vi "Dequeue.vi"(8 "error in (no error)":errorcluster caption="错误输入（无错误）", 11 "Queue 输入":refnum<class "Queue.lvclass"> caption="DNL_LabVIEW Object in") -> (0 "error out":errorcluster caption="错误输出", 2 "Item":variant, 3 "Queue 输出":refnum<class "Queue.lvclass"> caption="DNL_LabVIEW Object out")   [LabVIEW 2012, in "Queue.lvclass"]
uses:
  Queue.lvclass
  Queue.lvclass/Queue.ctl
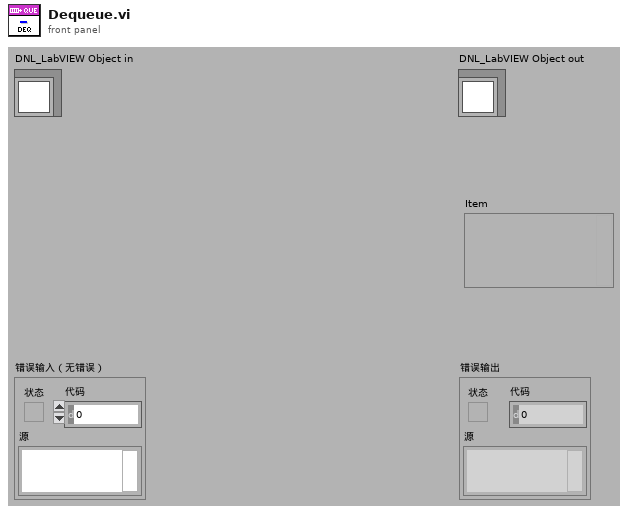
[diagram p1: front panel]
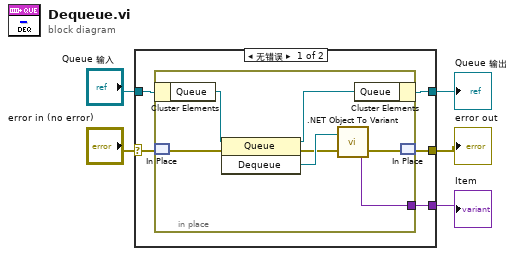
[diagram p0: block diagram]
diagram:
  n1 = case shown="无错误" "error in (no error)" {
    selector: "error in (no error)" -> [w8 w19]
    tunnel: [w7 w19] -> w4
    tunnel: [w9 w18] -> w2
    tunnel: "Queue 输入" -> [w10 w18]
    tunnel: [w6 _] -> w1
    frame No Error {
      n2 = in-place {
        in-place-border: [w11] -> w6
        n3 = in-place-cluster #1(w10) -> ("Queue"=w17:refnum<k24>)
        n4 = in-place-match #2(w8) -> (w15:errorcluster)
        n5 = invoke class="Queue" method="Dequeue"(reference=w17, error in=w15) -> (reference out=w16:refnum<k24>, error out=w13:errorcluster, "Dequeue"=w14:refnum<k24>)  [unwired: 1 in]
        n6 = call <vilib>:".NET Object To Variant.vi"("error in (no error)"=w13, ".NET object"=w14) -> ("error out"=w12:errorcluster, "variant"=w11:variant)
        n7 = in-place-cluster #1("Queue"=w16) -> (w9:refnum<class "Queue.lvclass">)
        n8 = in-place-match #2(w12) -> (w7:errorcluster)
      }
    }
    frame Error {
    }
  }
  "error out" <- w4
  "Queue 输出" <- w2
  "Item" <- w1
